vi "Fluence in Tile.vi"(0 "Analyze Fluence in":refnum<class "Analyze Fluence.lvclass">, 5 "Image in":T1, 11 "error in (no error)":errorcluster) -> (4 "Analyze Fluence out":refnum<class "Analyze Fluence.lvclass">, 6 "Image Dst Out":T1, 8 "Max Fluence":dbl[unit], 10 "fluence infos":T2[](array[typedef]), 15 "error out":errorcluster)   [LabVIEW 2014, in "Analyze.lvlib" / "Analyze Fluence.lvclass"]
uses:
  Analyze Fluence.lvclass
  Fluence Info.ctl
  <vilib>/vision/Image Controls.llb/IMAQ Image.ctl
  Analyze Parameter/Analyze Parameter Fluence/Analyze Parameter Fluence.lvclass
  Analyze Parameter/Analyze Parameter Energy/Analyze Parameter Energy.lvclass
  Analyze Fluence.lvclass/Analyze Fluence.ctl
  Analyze Parameter/Analyze Parameter Energy/Analyze Parameter Energy.lvclass/Analyze Parameter Energy.ctl
  <vilib>/vision/NI_Vision_Development_Module.lvlib
  Analyze BaseClass/Analyze BaseClass/Analyze BaseClass.lvclass
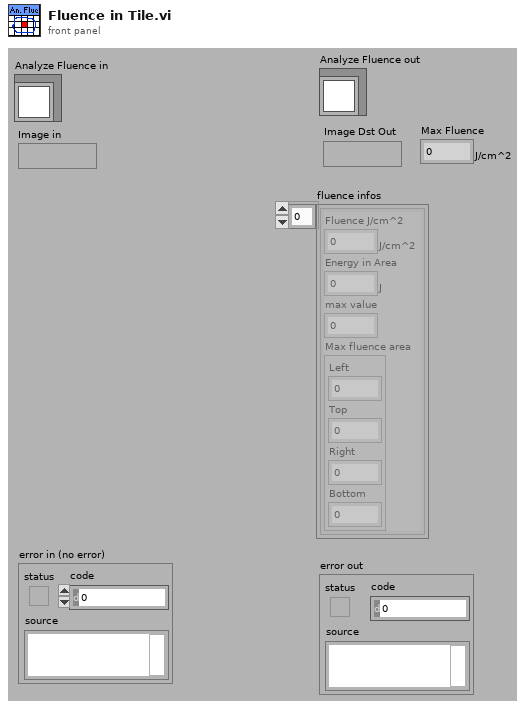
[diagram p1: front panel]
types:
  T1 = typedef "IMAQ Image.ctl" = refnum<image>
  T2 = typedef "Analyze.lvlib/Analyze Fluence.lvclass/Fluence Info.ctl" = cluster{"Fluence J/cm^2":dbl[unit], "Energy in Area":dbl[unit], "max value":i64, "Max fluence area":cluster{"Left":i32, "Top":i32, "Right":i32, "Bottom":i32}}
  T3 = cluster{"Left":i32, "Top":i32, "Right":i32, "Bottom":i32}
  T4 = typedef "Image Type" = u32
  T5 = typedef "ROI Descriptor" = cluster{"Global Rectangle":i32[], "Contours":cluster{"ID":enum32{"External", "Internal"}, "Type":u32, "Coordinates":i32[]}[]}
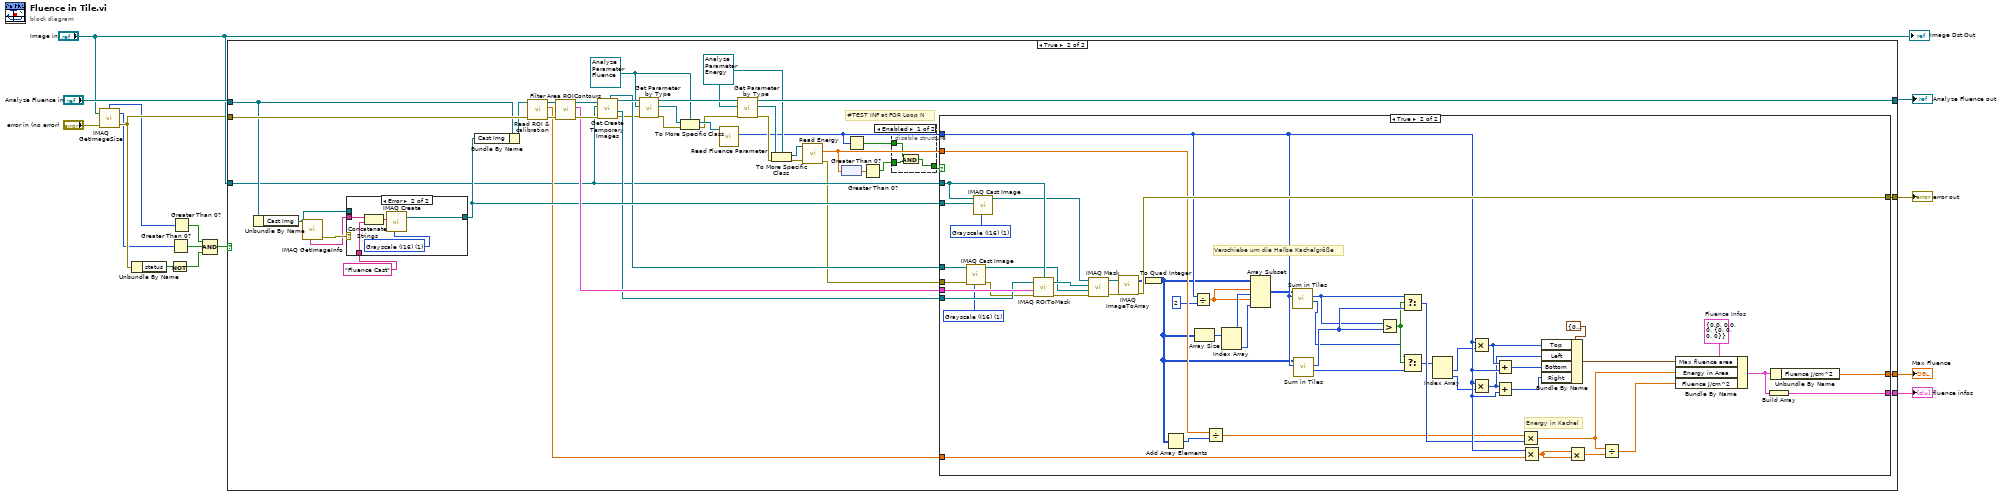
[diagram p0: block diagram]
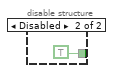
[diagram p3: hidden frame]
diagram:
  n1 = call "IMAQ GetImageSize"("Image"="Image in", "error in (no error)"="error in (no error)") -> ("Y Resolution"=w5:i32, "X Resolution"=w6:i32, "error out"=w8:errorcluster)  [unwired: 2 in]
  n2 = Unbundle By Name(w8) -> ("status"=w7:bool)
  n3 = Not(x=w7) -> (.not. x?=w2:bool)
  n4 = Greater Than 0?(x=w5) -> (x > 0?=w3:bool)
  n5 = Greater Than 0?(x=w6) -> (x > 0?=w4:bool)
  n6 = Compound Arithmetic op=AND(w4, w3, w2) -> (w1:bool)
  n7 = case shown="True" w1 {
    tunnel: [_ w58] -> w15
    tunnel: w8 -> [w16 w54]
    tunnel: "Analyze Fluence in" -> [w17 w50]
    tunnel: [w16 w40] -> w13
    tunnel: "Image in" -> [_ w39]
    tunnel: [_ w38] -> w12
    tunnel: [w17 w36] -> w11
    frame False {
    }
    frame True {
      w30 = refnum<class "Analyze Parameter Energy.lvclass"> refnum ("Energy")
      w33 = refnum<class "Analyze Parameter Fluence.lvclass"> refnum ("Parameter")
      # "#TEST INF at FOR Loop N"
      n8 = Unbundle By Name(w50) -> ("Cast Img"=w46:T1)
      n9 = call "IMAQ GetImageInfo"("Image"=w46) -> ("error out"=w49:errorcluster, "Image Name"=w48:string)  [unwired: 3 in, 6 out]
      n10 = case shown="Error" w49 {
        tunnel: w48 -> [_ w120]
        tunnel: "Fluence Cast" -> [_ w118]
        tunnel: [w116 w117] -> w44
        tunnel: w46 -> [w116 _]
        frame No Error {
        }
        frame Error {
          w121 = T4 1 items=["Grayscale (U8)", "Grayscale (I16)", "Grayscale (SGL)", "Complex (CSG)", "RGB (U32)", "HSL (U32)", "RGB (U64)", "Grayscale (U16)"] ("Image Type")
          n11 = Concatenate Strings(w120, w118) -> (w119:string)
          n12 = call "IMAQ Create"("Image Name"=w119, "Image Type"=w121) -> ("New Image"=w117:T1)  [unwired: 3 in, 1 out]
        }
      }
      n13 = Bundle By Name(cluster=w50, "Cast Img"=w44) -> (w45:refnum<class "Analyze Fluence.lvclass">)
      n14 = call-dynamic "Read ROI & calibration.vi"("error in (no error)"=w54, "Analyze BaseClass in"=w45) -> ("error out"=w53:errorcluster, "calibration mm/px"=w42:dbl[unit], "Analyze BaseClass out"=w56:refnum<class "Analyze Fluence.lvclass">)  [unwired: 6 in, 1 out]
      n15 = call-dynamic "Filter Area ROIContours.vi"("error in (no error)"=w53, "Analyze BaseClass in"=w56) -> ("error out"=w52:errorcluster, "ROI of Area type"=w51:T5, "Analyze BaseClass out"=w55:refnum<class "Analyze Fluence.lvclass">)  [unwired: 7 in]
      n16 = call-dynamic "Get Create Temporary Images.vi"("error in (no error)"=w52, "Image in"=w39, "Analyze BaseClass in"=w55) -> ("error out"=w25:errorcluster, "image mask"=w41:T1, "Analyze BaseClass out"=w57:refnum<class "Analyze Fluence.lvclass">, "masked image"=w43:T1)  [unwired: 4 in, 1 out]
      n17 = call "Get Parameter by Type.vi"("error in (no error)"=w25, "Parameter Type"=w33, "Analyze BaseClass in"=w57) -> ("error out"=w29:errorcluster, "Parameter"=w35:refnum<class "Analyze Parameter Base.lvclass">, "Analyze BaseClass out"=w37:refnum<class "Analyze Fluence.lvclass">)  [unwired: 5 in, 1 out]
      n18 = To More Specific Class(target class=w33, reference=w35, error in=w29) -> (specific class reference=w34:refnum<class "Analyze Parameter Fluence.lvclass">, error out=w28:errorcluster)
      n19 = call "Read Fluence Parameter.vi"("Analyze Parameter Fluence in"=w34) -> ("Size of region (px)"=w23:i32)  [unwired: 7 in, 3 out]
      n20 = call "Get Parameter by Type.vi"("error in (no error)"=w28, "Parameter Type"=w30, "Analyze BaseClass in"=w37) -> ("error out"=w27:errorcluster, "Parameter"=w31:refnum<class "Analyze Parameter Base.lvclass">, "Analyze BaseClass out"=w36:refnum<class "Analyze Fluence.lvclass">)  [unwired: 5 in, 1 out]
      n21 = To More Specific Class(target class=w30, reference=w31, error in=w27) -> (specific class reference=w32:refnum<class "Analyze Parameter Energy.lvclass">, error out=w26:errorcluster)
      n22 = call "Read Energy.vi"("error in (no error)"=w26, "Analyze Parameter Energy in"=w32) -> ("error out"=w24:errorcluster, "Energy"=w22:dbl[unit])  [unwired: 7 in, 1 out]
      n23 = node(w22) -> (w21:dbl)
      n24 = Greater Than 0?(x=w23) -> (x > 0?=w20:bool)
      n25 = Greater Than 0?(x=w21) -> (x > 0?=w19:bool)
      n26 = disable-structure shown="Enabled" {
        disable-tunnel: w20 -> [w61 _]
        disable-tunnel: w19 -> [w60 _]
        disable-tunnel: [w59 TRUE] -> w18
        frame Enabled {
          n27 = And(x=w61, y=w60) -> (x .and. y?=w59:bool)
        }
        frame Disabled {
        }
      }
      n28 = case shown="True" w18 {
        tunnel: [_ w115] -> w58
        tunnel: w51 -> [_ w114]
        tunnel: w44 -> [_ w113]
        tunnel: w43 -> [_ w112]
        tunnel: w42 -> [_ w111]
        tunnel: w41 -> [_ w110]
        tunnel: [w63 w109] -> w40
        tunnel: w39 -> [_ w108]
        tunnel: [_ w107] -> w38
        tunnel: w23 -> [_ w106]
        tunnel: w22 -> [_ w105]
        tunnel: w24 -> [w63 w104]
        frame False {
        }
        frame True {
          w69 = T2 {"Fluence J/cm^2"=0.0, "Energy in Area"=0.0, "max value"=0, "Max fluence area"={"Left"=0, "Top"=0, "Right"=0, "Bottom"=0}}  # Fluence Infos
          w96 = T4 1 items=["Grayscale (U8)", "Grayscale (I16)", "Grayscale (SGL)", "Complex (CSG)", "RGB (U32)", "HSL (U32)", "RGB (U64)", "Grayscale (U16)"] ("Image Type")
          w98 = T4 1 items=["Grayscale (U8)", "Grayscale (I16)", "Grayscale (SGL)", "Complex (CSG)", "RGB (U32)", "HSL (U32)", "RGB (U64)", "Grayscale (U16)"] ("Image Type")
          # "Verschiebe um die Halbe Kachelgröße"
          # "Energy in Kachel"
          n29 = call "IMAQ Cast Image"("Image Type"=w96, "error in (no error)"=w104, "Image Src"=w112) -> ("error out"=w95:errorcluster, "Image Dst Out"=w97:T1)  [unwired: 7 in]
          n30 = call "IMAQ Cast Image"("Image Type"=w98, "Image Dst"=w113, "Image Src"=w108) -> ("Image Dst Out"=w99:T1)  [unwired: 7 in, 1 out]
          n31 = call "IMAQ ROIToMask"("error in (no error)"=w95, "ROI Descriptor"=w114, "Image"=w110, "Image Model"=w108) -> ("error out"=w102:errorcluster, "Image Out"=w103:T1)  [unwired: 2 in, 1 out]
          n32 = call "IMAQ Mask"("error in (no error)"=w102, "Image Dst"=w97, "Image Mask"=w103, "Image Src"=w99) -> ("error out"=w81:errorcluster, "Image Dst Out"=w82:T1)  [unwired: 1 in]
          n33 = call "IMAQ ImageToArray"("error in (no error)"=w81, "Image"=w82) -> ("error out"=w109:errorcluster, "Image Pixels (I16)"=w101:i16[][])  [unwired: 2 in, 3 out]
          n34 = To Quad Integer(1:w101) -> (0:w100:i64[][])
          n35 = Add Array Elements(numeric array=w100) -> (sum=w94:i64)
          n36 = Divide(x=w106, y=2 ("x")) -> (x/y=w87:dbl)
          n37 = Array Size(array=w100) -> (size(s)=w88:i32[])
          n38 = Divide(x=w105, y=w94) -> (x/y=w84:dbl[unit])
          n39 = Index Array(array=w88) -> (element #1=w89:i32, element #2=w90:i32)  [unwired: 2 in]
          n40 = Array Subset(array=w100, index (row)=w87, length (row)=w89, index (col)=w87, length (col)=w90) -> (w91:i64[][])
          n41 = call "Sum in Tiles.vi"("size"=w106, "Image"=w91) -> ("Max Index"=w78:i32[], "Maximum"=w92:i64)  [unwired: 7 in, 1 out]
          n42 = call "Sum in Tiles.vi"("size"=w106, "Image"=w100) -> ("Max Index"=w77:i32[], "Maximum"=w93:i64)  [unwired: 7 in, 1 out]
          n43 = Greater?(x=w92, y=w93) -> (0:w79:bool)
          n44 = Select(t=w92, s=w79, f=w93) -> (s? t:f=w85:i64)
          n45 = Select(t=w78, s=w79, f=w77) -> (s? t:f=w76:i32[])
          n46 = Index Array(array=w76) -> (element #1=w75:i32, element #2=w74:i32)  [unwired: 2 in]
          n47 = Multiply(x=w106, y=w75) -> (x*y=w71:i32)
          n48 = Multiply(x=w106, y=w74) -> (x*y=w70:i32)
          n49 = Add(x=w71, y=w106) -> (x+y=w72:i32)
          n50 = Add(x=w70, y=w106) -> (x+y=w73:i32)
          n51 = Multiply(x=w84, y=w85) -> (x*y=w67:dbl[unit])
          n52 = Multiply(x=w106, y=w111) -> (x*y=w64:dbl[unit])
          n53 = Bundle By Name(cluster=T3 {"Left"=0, "Top"=0, "Right"=0, "Bottom"=0} ("Rectangle"), "Top"=w71, "Left"=w70, "Bottom"=w72, "Right"=w73) -> (w68:T3)
          n54 = Multiply(x=w64, y=w64) -> (x*y=w83:dbl[unit])
          n55 = Divide(x=w67, y=w83) -> (x/y=w66:dbl[unit])
          n56 = Bundle By Name(cluster=w69, "Max fluence area"=w68, "Energy in Area"=w67, "Fluence J/cm^2"=w66) -> (w65:T2)
          n57 = Build Array(w65) -> (w107:T2[])
          n58 = Unbundle By Name(w65) -> ("Fluence J/cm^2"=w115:dbl[unit])
        }
      }
    }
  }
  "fluence infos" <- w12
  "error out" <- w13
  "Max Fluence" <- w15
  "Analyze Fluence out" <- w11
  "Image Dst Out" <- "Image in"
